vi "Outputs SW Set.vi"(7 "Current Time":timestamp format="%<%x %.3X>T", 8 "Wrist Config":T1={"WristHW Ver"=0, "CAN"={"ID"=0, "Bus"=""}, "Output"={"Type"=enum."Counter-Clockwise", "Neutral"=enum."Override to Coast", "Max"={"FWD"=1.0, "REV"=-1.0}, "Min"={"FWD"=0.0, "REV"=0.0}, "OL Ramp Rate (S)"=0.0, "Dead Band"=0.0}, "CL"={"Gains"={"P"=1.0, "I"=0.01, "D"=0.0, "F"=0.0}, "Error Allowed"={"High"=0.0, "Low"=0.0}, "I Zone"={"High"=10000.0, "Low"=-1000.0}, "Max Out"={"FWD"=1.0, "REV"=-1.0}, "Max I Accu"={"High"=10.0, "Low"=-10.0}, "CL Ramp Rate (S)"=0.0}, "MM"={"Cruise Velocity"=5000, "Acceleration"=5000}, "TravelLimits"={"Hard"={"FWD Switch Normal"=enum."Normally Open", "FWD On will Zero Encoder "=FALSE, "REV Switch Normal"=enum."Normally Open", "REV On will Zero Encoder "=FALSE}, "Soft"={"FWD"={"Enable"=FALSE, "Counts"=0}, "REV"={"Enable"=FALSE, "Counts"=0}}}, "Cancoder"={"ID"=0, "CW(t) CCW(f)"=TRUE, "Zero Offset"=0.0}, "CurrentLimit"={"Enable"=FALSE, "Current Limit"=0.0, "Threshold Current"=0.0, "Threshold Time"=0.0}} {"TravelLimits"."Soft"."REV"."Counts" format="%#.0f"; "TravelLimits"."Soft"."FWD"."Counts" format="%#.0f"; "Output"."Min"."REV" format="%.2f"; "Output"."Min"."FWD" format="%.2f"; "Output"."Max"."REV" format="%.2f"; "Output"."Max"."FWD" format="%.2f"; "CL"."Max I Accu"."Low" format="%#.8f"; "CL"."Max I Accu"."High" format="%#.8f"; "CL"."Gains"."F" format="%#.8f"; "CL"."Gains"."D" format="%#.8f"; "CL"."Gains"."I" format="%#.8f"; "CL"."Gains"."P" format="%#.8f"; "CL"."Error Allowed"."Low" format="%#.8f"; "CL"."Error Allowed"."High" format="%#.8f"; "CL"."I Zone"."Low" format="%#.8f"; "CL"."I Zone"."High" format="%#.8f"; "CL"."Max Out"."REV" format="%.2f"; "CL"."Max Out"."FWD" format="%.2f"}, 9 "WristSW Config":T18={"WristSW Ver"=0, "At Position Delay(S)"=0.2}, 10 "Sensor Values":T20, 11 "SW Output":T19) -> (3 "SW Output Out":T19)   [LabVIEW 2020, in "Wrist_ACT.lvlib"]
uses:
  Wrist_ACT.lvlib
  Shared Code/TypeDefs/Cluster_Wrist HW Outputs.ctl
  Shared Code/TypeDefs/Cluster_FX Sensor Values.ctl
  Shared Code/TypeDefs/Cluster_FX CloseLoop Values.ctl
  Shared Code/TypeDefs/Cluster_FX Limit Switchs.ctl
  Shared Code/TypeDefs/Cluster_FX Current Values.ctl
  Shared Code/TypeDefs/Cluster_FX Integrated Sensor Values.ctl
  Shared Code/TypeDefs/Cluster_Wrist_SW Output Data.ctl
  Shared Code/TypeDefs/Cluster_Wrist_Config SW Values.ctl
  Shared Code/TypeDefs/Cluster_Wrist_Config HW Values.ctl
  Shared Code/TypeDefs/Cluser_CAN Data.ctl
  Shared Code/TypeDefs/Cluster_Config Motor Output.ctl
  <vilib>/Rock Robotics/WPI/ThirdParty/Phoenix-LabVIEW/Motor Controller/Controls/CTRE_Phoenix_MotorControl_TalonFXInvertType.ctl
  <vilib>/Rock Robotics/WPI/ThirdParty/Phoenix-LabVIEW/Motor Controller/Controls/CTRE_Phoenix_MotorControl_NeutralMode.ctl
  Shared Code/TypeDefs/Cluster_FWD  REV Values.ctl
  Shared Code/TypeDefs/Cluster_PID Config.ctl
  Shared Code/TypeDefs/Cluster_PID Gains.ctl
  Shared Code/TypeDefs/Cluster_High-Low.ctl
  Shared Code/TypeDefs/Cluster_Motion Magic Parameters.ctl
  Shared Code/TypeDefs/Cluser_Limit Travel Config.ctl
  Shared Code/TypeDefs/Cluser_Hard Limits.ctl
  <vilib>/Rock Robotics/WPI/ThirdParty/Phoenix-LabVIEW/Motor Controller/Controls/CTRE_Phoenix_MotorControl_LimitSwitchNormal.ctl
  Shared Code/TypeDefs/Cluser_Config_Soft Limits.ctl
  Shared Code/TypeDefs/Cluser_Enable-Value I32.ctl
  Shared Code/TypeDefs/Cluster_Config_Cancoder Data.ctl
  Shared Code/TypeDefs/Cluser_Config_Current Limits.ctl
panel:
  # "Tune Output\nto 1023 Max"
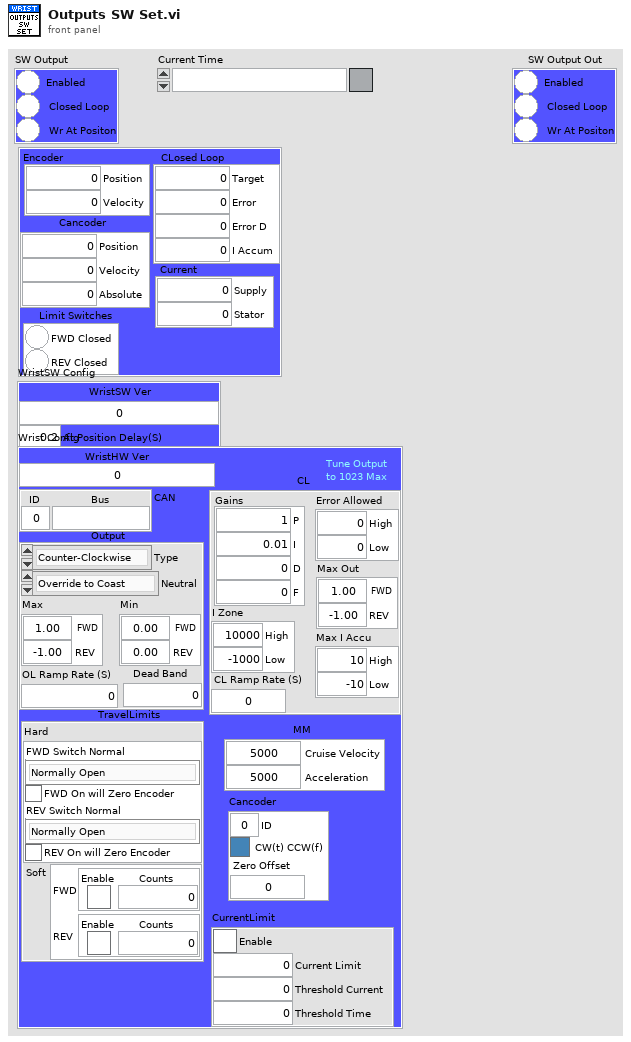
[diagram p1: front panel]
types:
  T1 = typedef "Cluster_Wrist_Config HW Values.ctl" = cluster{"WristHW Ver":u64, "CAN":T2, "Output":T3, "CL":T7, "MM":T10, "TravelLimits":T11, "Cancoder":T16, "CurrentLimit":T17}
  T2 = typedef "Cluser_CAN Data.ctl" = cluster{"ID":u8, "Bus":string}
  T3 = typedef "Cluster_Config Motor Output.ctl" = cluster{"Type":T4, "Neutral":T5, "Max":T6, "Min":T6, "OL Ramp Rate (S)":dbl, "Dead Band":dbl}
  T4 = typedef "CTRE_Phoenix_MotorControl_TalonFXInvertType.ctl" = enum16{"Counter-Clockwise", "Clockwise"}
  T5 = typedef "CTRE_Phoenix_MotorControl_NeutralMode.ctl" = enum8{"EEPROMSetting", "Override to Coast", "Override to Brake"}
  T6 = typedef "Cluster_FWD  REV Values.ctl" = cluster{"FWD":dbl, "REV":dbl}
  T7 = typedef "Cluster_PID Config.ctl" = cluster{"Gains":T8, "Error Allowed":T9, "I Zone":T9, "Max Out":T6, "Max I Accu":T9, "CL Ramp Rate (S)":dbl}
  T8 = typedef "Cluster_PID Gains.ctl" = cluster{"P":dbl, "I":dbl, "D":dbl, "F":dbl}
  T9 = typedef "Cluster_High-Low.ctl" = cluster{"High":dbl, "Low":dbl}
  T10 = typedef "Cluster_Motion Magic Parameters.ctl" = cluster{"Cruise Velocity":i32, "Acceleration":i32}
  T11 = typedef "Cluser_Limit Travel Config.ctl" = cluster{"Hard":T12, "Soft":T14}
  T12 = typedef "Cluser_Hard Limits.ctl" = cluster{"FWD Switch Normal":T13, "FWD On will Zero Encoder ":bool, "REV Switch Normal":T13, "REV On will Zero Encoder ":bool}
  T13 = typedef "CTRE_Phoenix_MotorControl_LimitSwitchNormal.ctl" = enum16{"Normally Open", "Normally Closed", "Disabled"}
  T14 = typedef "Cluser_Config_Soft Limits.ctl" = cluster{"FWD":T15, "REV":T15}
  T15 = typedef "Cluser_Enable-Value I32.ctl" = cluster{"Enable":bool, "Counts":i32}
  T16 = typedef "Cluster_Config_Cancoder Data.ctl" = cluster{"ID":u8, "CW(t) CCW(f)":bool, "Zero Offset":dbl}
  T17 = typedef "Cluser_Config_Current Limits.ctl" = cluster{"Enable":bool, "Current Limit":dbl, "Threshold Current":dbl, "Threshold Time":dbl}
  T18 = typedef "Cluster_Wrist_Config SW Values.ctl" = cluster{"WristSW Ver":u64, "At Position Delay(S)":dbl}
  T19 = typedef "Cluster_Wrist_SW Output Data.ctl" = cluster{"Enabled":bool, "Closed Loop":bool, "Wr At Positon":bool}
  T20 = typedef "Cluster_Wrist HW Outputs.ctl" = cluster{"Encoder":T21, "CLosed Loop":T22, "Limit Switches":T23, "Current":T24, "Cancoder":T25}
  T21 = typedef "Cluster_FX Sensor Values.ctl" = cluster{"Position":i32, "Velocity":i32}
  T22 = typedef "Cluster_FX CloseLoop Values.ctl" = cluster{"Target":dbl, "Error":i32, "Error D":dbl, "I Accum":dbl}
  T23 = typedef "Cluster_FX Limit Switchs.ctl" = cluster{"FWD Closed":bool, "REV Closed":bool}
  T24 = typedef "Cluster_FX Current Values.ctl" = cluster{"Supply":dbl, "Stator":dbl}
  T25 = typedef "Cluster_FX Integrated Sensor Values.ctl" = cluster{"Position":dbl, "Velocity":dbl, "Absolute":dbl}
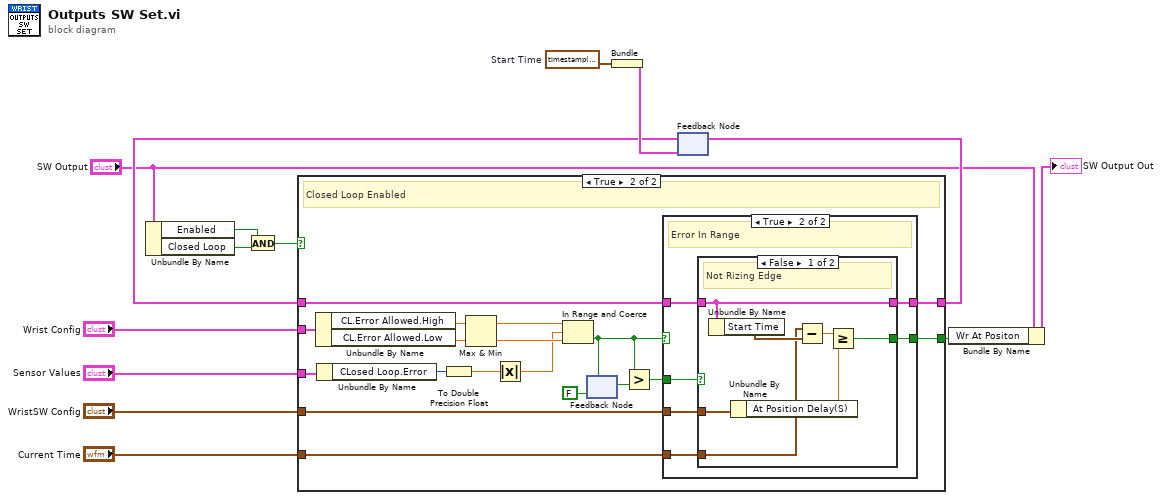
[diagram p0: block diagram]
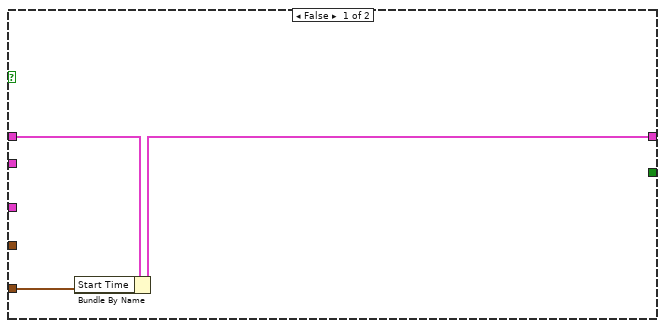
[diagram p2: hidden frame]
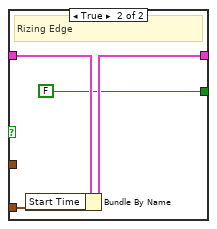
[diagram p4: hidden frame]
diagram:
  w8 = timestamp(0 s since 1904-01-01)  # Start Time
  n1 = Unbundle By Name("SW Output") -> ("Enabled"=w14:bool, "Closed Loop"=w13:bool)
  n2 = And(x=w14, y=w13) -> (x .and. y?=w9:bool)
  n3 = Bundle("Start Time"=w8) -> (w7:cluster{"Start Time":timestamp})  [unwired: 1 in]
  n4 = feedback #1(w7) -> (w6:cluster{"Start Time":timestamp})
  n5 = case shown="True" w9 {
    tunnel: "WristSW Config" -> [_ w35]
    tunnel: "Sensor Values" -> [_ w33]
    tunnel: "Current Time" -> [w16 w24]
    tunnel: w6 -> [w17 w34]
    tunnel: [w15 w25] -> w5
    tunnel: [_ w23] -> w2
    tunnel: "Wrist Config" -> [_ w32]
    frame False {
      n6 = Bundle By Name(cluster=w17, "Start Time"=w16) -> (w15:cluster{"Start Time":timestamp})
    }
    frame True {
      # "Closed Loop Enabled"
      n7 = Unbundle By Name(w32) -> ("CL.Error Allowed.High"=w22:dbl, "CL.Error Allowed.Low"=w20:dbl)
      n8 = Unbundle By Name(w33) -> ("CLosed Loop.Error"=w31:i32)
      n9 = To Double Precision Float(number=w31) -> (double precision float=w30:dbl)
      n10 = Max & Min(x=w22, y=w20) -> (max(x,y)=w21:dbl, min(x,y)=w19:dbl)
      n11 = Absolute Value(x=w30) -> (abs(x)=w18:dbl)
      n12 = In Range and Coerce(upper limit=w21, x=w18, lower limit=w19) -> (In Range?=w27:bool)  [unwired: 1 out]
      n13 = feedback #2(FALSE) -> (w29:bool)
      n14 = feedback-in #2(w27) -> ()
      n15 = Greater?(x=w27, y=w29) -> (0:w26:bool)
      n16 = case shown="True" w27 {
        selector: w27 -> [w36 _]
        tunnel: w35 -> [_ w43]
        tunnel: w34 -> [w37 w41]
        tunnel: w26 -> [_ w42]
        tunnel: [w37 w40] -> w25
        tunnel: w24 -> [_ w39]
        tunnel: [w36 w38] -> w23
        frame False {
          # "Error Out of Range"
        }
        frame True {
          # "Error In Range"
          n17 = case shown="False" w42 {
            tunnel: w43 -> [w46 _]
            tunnel: w41 -> [w50 w52]
            tunnel: [w50 w53] -> w40
            tunnel: w39 -> [w48 w54]
            tunnel: [w44 FALSE] -> w38
            frame False {
              # "Not Rizing Edge"
              n18 = Unbundle By Name(w50) -> ("Start Time"=w49:timestamp)
              n19 = Unbundle By Name(w46) -> ("At Position Delay(S)"=w45:dbl)
              n20 = Subtract(x=w48, y=w49) -> (x-y=w47:dbl)
              n21 = Greater Or Equal?(x=w47, y=w45) -> (x >= y?=w44:bool)
            }
            frame True {
              # "Rizing Edge"
              n22 = Bundle By Name(cluster=w52, "Start Time"=w54) -> (w53:cluster{"Start Time":timestamp})
            }
          }
        }
      }
    }
  }
  n23 = feedback-in #1(w5) -> ()
  n24 = Bundle By Name(cluster="SW Output", "Wr At Positon"=w2) -> (→"SW Output Out":T19)
